vi "minicryo_SequenceRunner_202102.vi"() -> ()   [LabVIEW 2013]
uses:
  B_Globals.vi
  Global 2.vi
  DeltaRamp_globals.vi
panel:
  out "Output File":path=path "C:/User Data/Guang/EuS junction/EJJ 008D/JJ7_RH_8-10-14-1/RH_10uA_10K.txt"
  in  "Directory":path=path "C:/User Data/Guang/EuS junction/EJJ 008D/JJ7_RH_8-10-14-1"
  in  "T_high":dbl
  in  "T_low":dbl
  in  "Skip":bool
  out "Step":dbl
  out "Of":dbl=1.0
  out "Action":string="Waiting for go"
  in  "Start":bool
  in  "Array":T1(array[cluster])=[{"Combo Box"="Start R(H) (Bundle)", "Rate"=0.1, "Set Point"=-0.5, "String"="RH_10uA_10K", "Step [T]"=0.0, "Settle [s]"=0.0}]
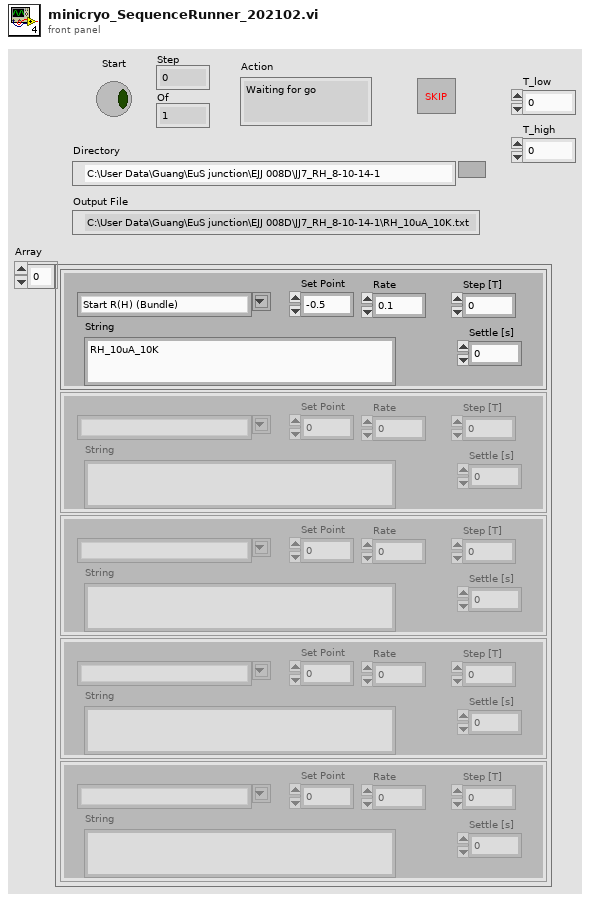
[diagram p1: front panel]
types:
  T1 = cluster{"Combo Box":string, "Rate":dbl, "Set Point":dbl, "String":string, "Step [T]":dbl, "Settle [s]":dbl}[]
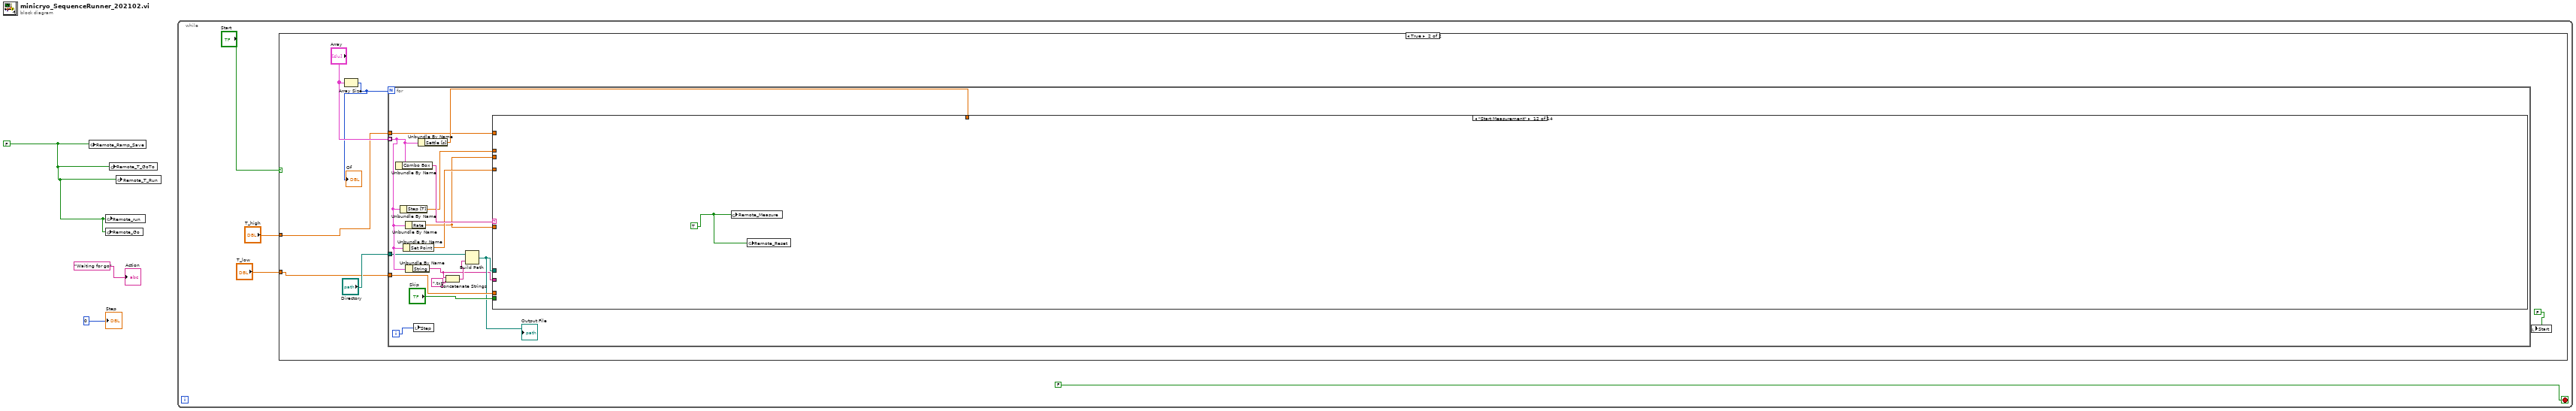
[diagram p0: block diagram]
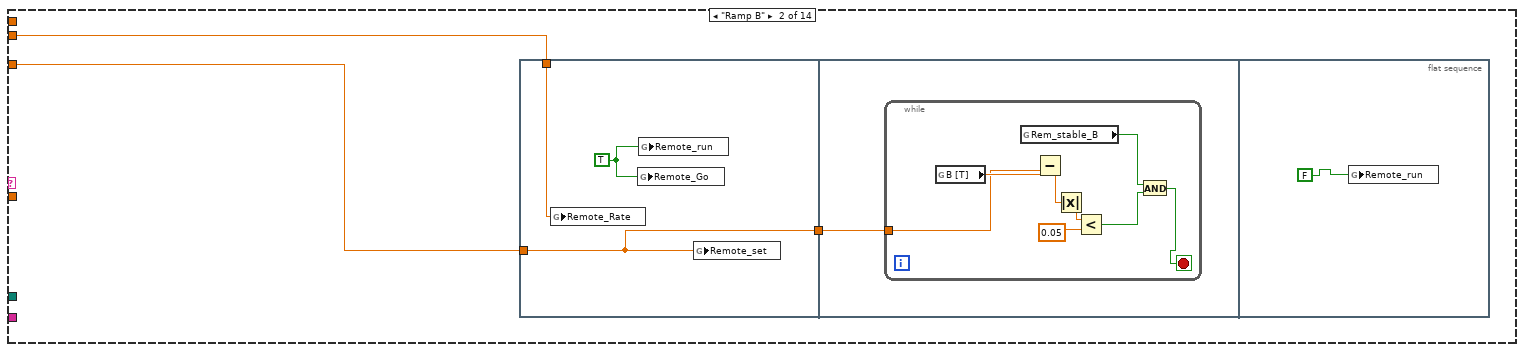
[diagram p4: hidden frame]
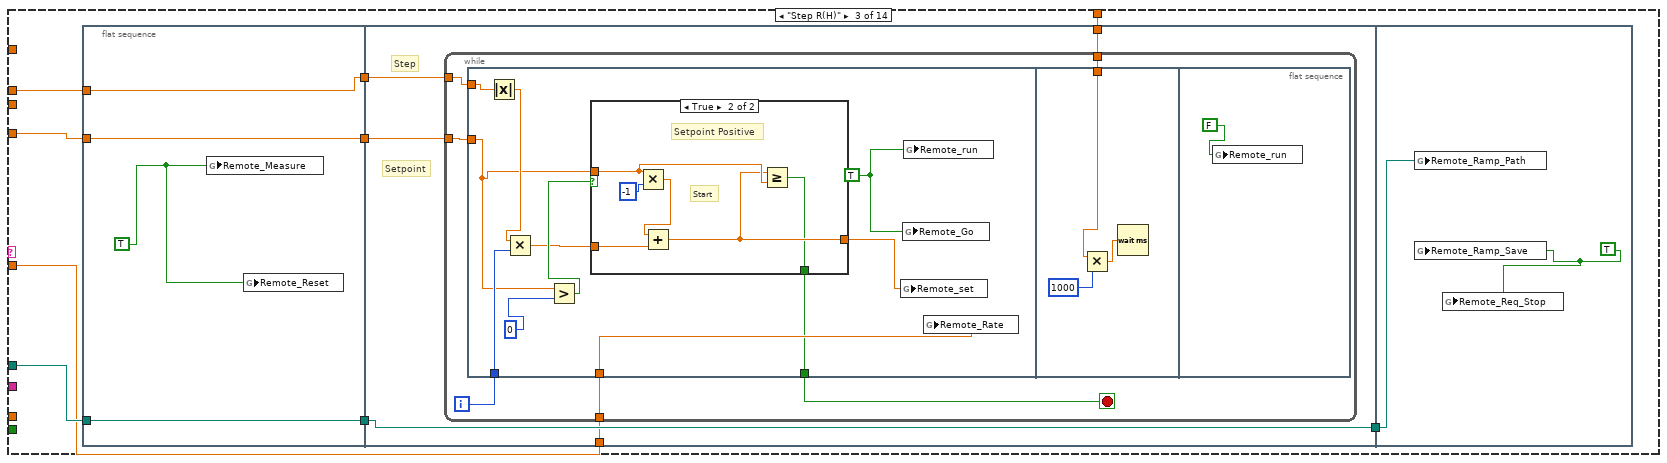
[diagram p5: hidden frame]
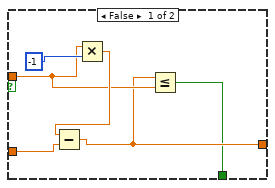
[diagram p6: hidden frame]
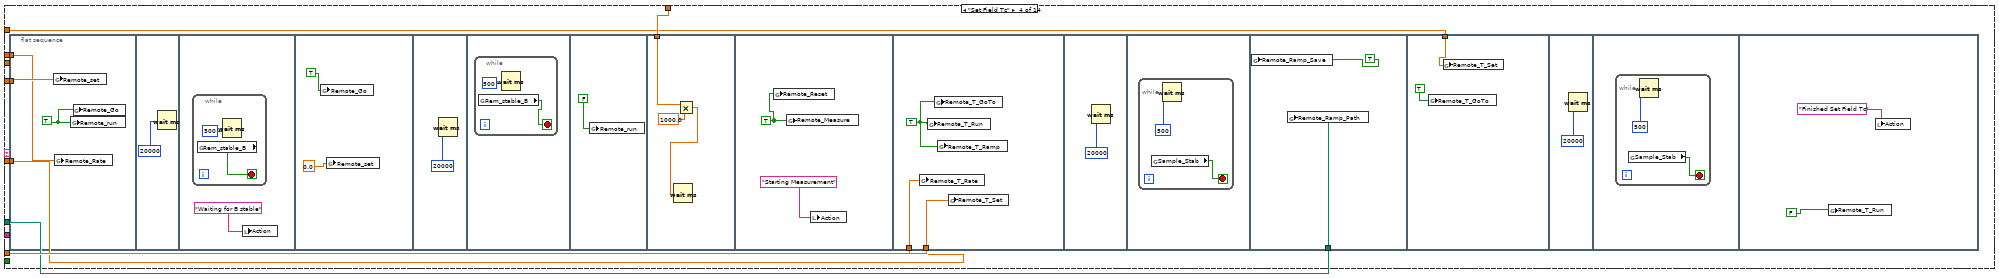
[diagram p7: hidden frame]
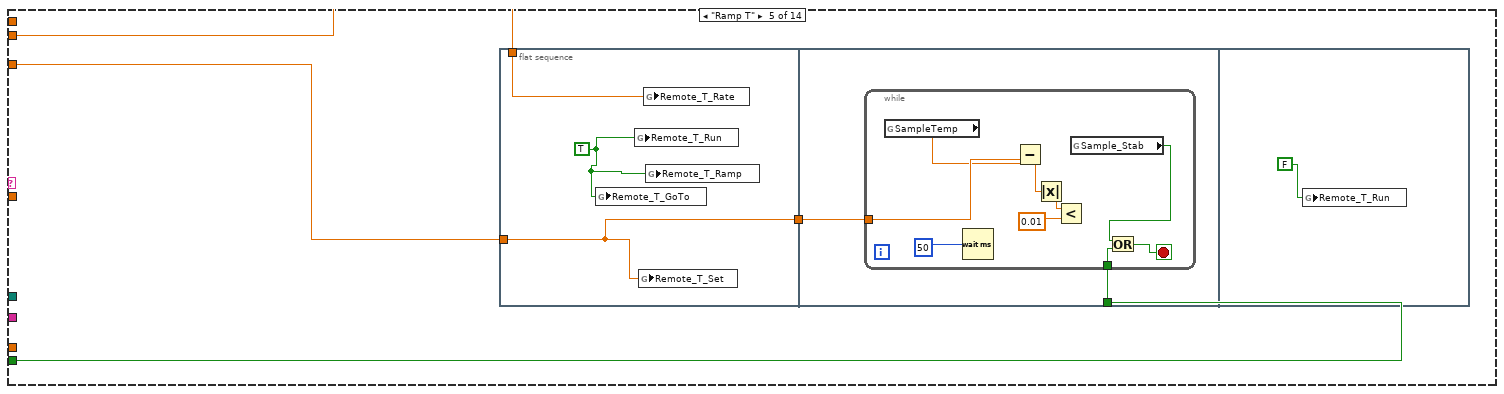
[diagram p8: hidden frame]
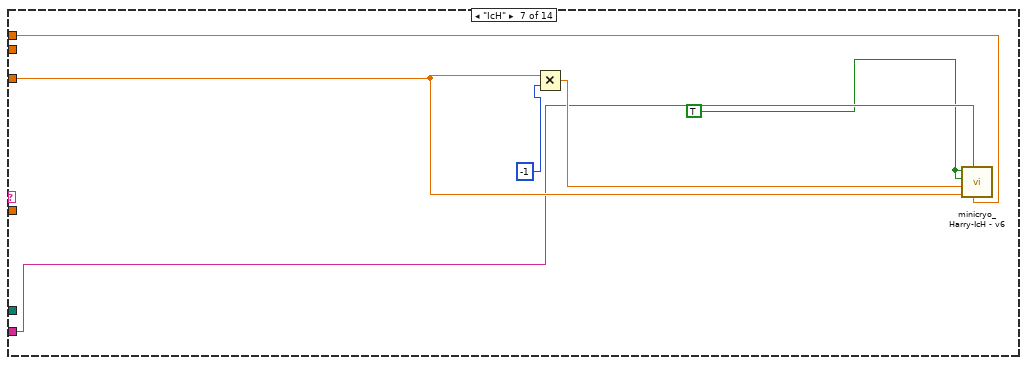
[diagram p10: hidden frame]
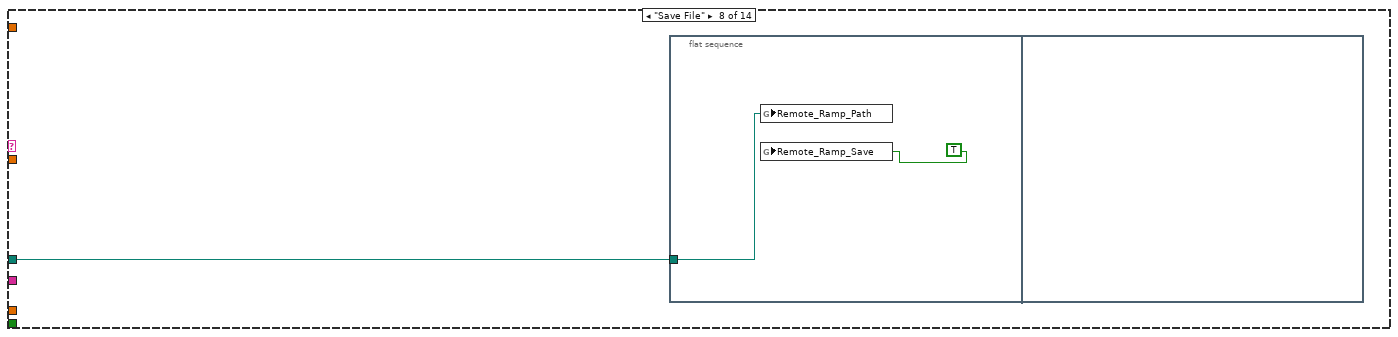
[diagram p11: hidden frame]
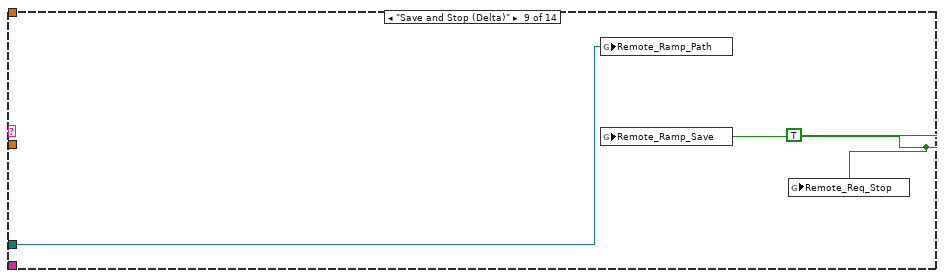
[diagram p12: hidden frame]
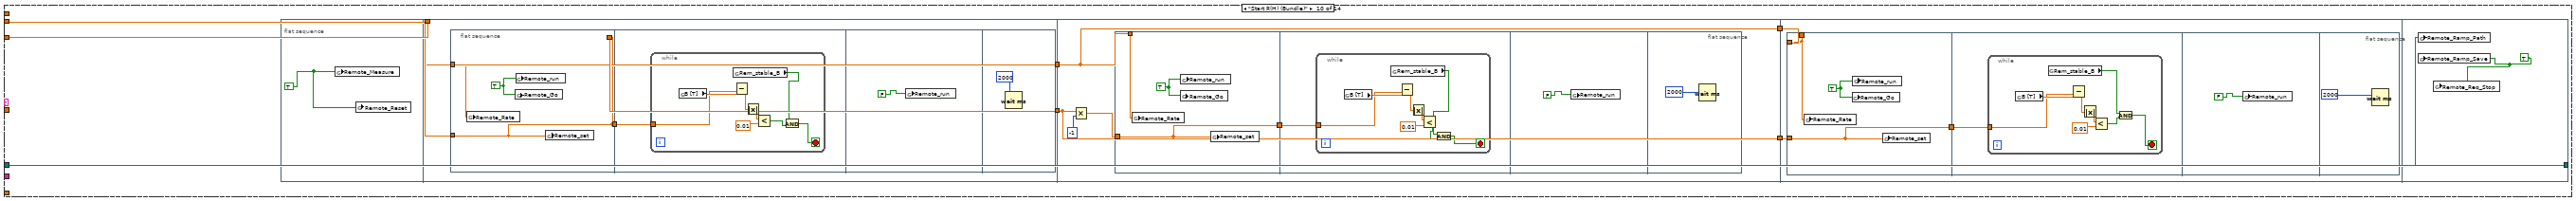
[diagram p13: hidden frame]
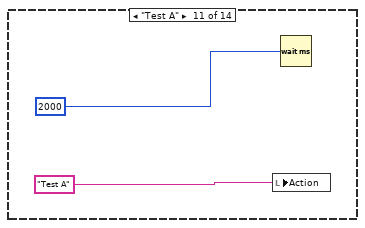
[diagram p14: hidden frame]
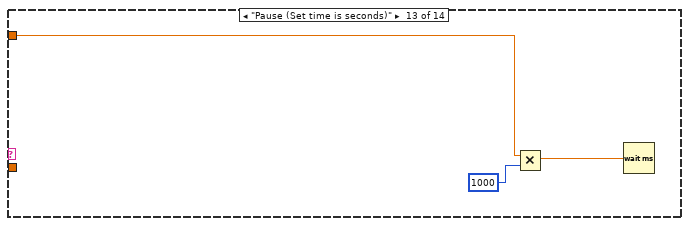
[diagram p15: hidden frame]
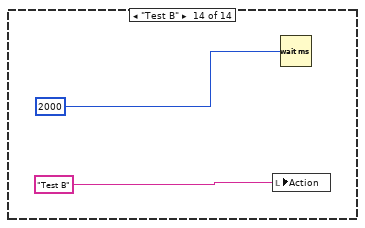
[diagram p16: hidden frame]
diagram:
  w3 = FALSE
  n1 = global write "DeltaRamp_globals.vi" "Remote_Ramp_Save"(w3) -> ()
  n2 = global write "B_Globals.vi" "Remote_Go"(w3) -> ()
  n3 = global write "B_Globals.vi" "Remote_run"(w3) -> ()
  n4 = global write "Global 2.vi" "Remote_T_GoTo"(w3) -> ()
  n5 = global write "Global 2.vi" "Remote_T_Run"(w3) -> ()
  n6 = while {
    stop <- FALSE stop-if-true
    n7 = case shown="True" "Start" {
      tunnel: "T_high" -> [_ w8]
      tunnel: "T_low" -> [_ w9]
      frame False {
      }
      frame True {
        n8 = Array Size(array="Array") -> (size(s)=w11:i32)
        "Of" <- w11
        n9 = for {
          N: w11 -> [_]
          tunnel: "Array" -> [w24] mode=indexing
          tunnel: "Directory" -> [w20]
          tunnel: w9 -> [w17]
          tunnel: w8 -> [w16]
          i -> [w26]
          n10 = Unbundle By Name(w24) -> ("Combo Box"=w28:string)
          n11 = Unbundle By Name(w24) -> ("Step [T]"=w22:dbl)
          n12 = Unbundle By Name(w24) -> ("Set Point"=w27:dbl)
          n13 = Unbundle By Name(w24) -> ("Rate"=w21:dbl)
          n14 = Unbundle By Name(w24) -> ("String"=w14:string)
          n15 = local write "Step"(w26) -> ()
          n16 = Unbundle By Name(w24) -> ("Settle [s]"=w23:dbl)
          n17 = Concatenate Strings(w14, ".txt") -> (w18:string)
          n18 = Build Path(base path=w20, name or relative path=w18) -> (appended path=w15:path)
          "Output File" <- w15
          n19 = case shown="\"Start Measurement\"" w28 {
            tunnel: w27 -> [_ w31 w49 w104 w139 _ w160 _ _ w174 _ _ w236 _]
            tunnel: w21 -> [_ w30 _ _ w140 _ _ _ _ w173 _ _ _ _]
            tunnel: w15 -> [_ _ w52 w99 _ _ _ w163 w167 w168 _ _ _ _]
            tunnel: "Skip" -> [_ _ _ _ w138 _ _ _ _ _ _ _ _ _]
            tunnel: w23 -> [_ _ w47 w103 _ _ _ _ _ _ _ _ _ _]
            tunnel: w22 -> [_ _ w46 w98 _ _ w159 _ _ _ _ _ _ _]
            tunnel: w21 -> [_ _ w45 w101 _ _ _ _ _ _ _ _ _ _]
            tunnel: w17 -> [_ _ _ w102 _ _ _ _ _ _ _ _ _ _]
            tunnel: w16 -> [_ _ _ w100 _ _ _ _ _ _ _ _ _ _]
            tunnel: w14 -> [_ _ _ _ _ _ w158 _ _ _ _ _ _ _]
            frame "False", Default {
            }
            frame "Ramp B" {
              n20 = flat-sequence {
                tunnel: w31 -> [w32]
                tunnel: w30 -> [w33]
                tunnel: [w32] -> w29
                tunnel: w29 -> [w35]
                frame #0 {
                  w34 = TRUE
                  n21 = global write "B_Globals.vi" "Remote_Rate"(w33) -> ()
                  n22 = global write "B_Globals.vi" "Remote_Go"(w34) -> ()
                  n23 = global write "B_Globals.vi" "Remote_run"(w34) -> ()
                  n24 = global write "B_Globals.vi" "Remote_set"(w32) -> ()
                }
                frame #1 {
                  n25 = while {
                    tunnel: w35 -> [w42]
                    stop <- w36 stop-if-true
                    n26 = global read "B_Globals.vi" "B [T]"() -> (w43:dbl)
                    n27 = global read "B_Globals.vi" "Rem_stable_B"() -> (w38:bool)
                    n28 = Subtract(x=w43, y=w42) -> (x-y=w41:dbl)
                    n29 = Absolute Value(x=w41) -> (abs(x)=w40:dbl)
                    n30 = Less?(x=w40, y=0.05) -> (x < y?=w37:bool)
                    n31 = And(x=w38, y=w37) -> (x .and. y?=w36:bool)
                  }
                }
                frame #2 {
                  n32 = global write "B_Globals.vi" "Remote_run"(FALSE) -> ()
                }
              }
            }
            frame "Step R(H)" {
              n33 = flat-sequence {
                tunnel: [w56] -> w53
                tunnel: w52 -> [w56]
                tunnel: [w55] -> w50
                tunnel: w49 -> [w55]
                tunnel: [w54] -> w48
                tunnel: w46 -> [w54]
                tunnel: w53 -> [w62]
                tunnel: [w62] -> w51
                tunnel: w50 -> [w61]
                tunnel: w48 -> [w60]
                tunnel: w47 -> [w59]
                tunnel: w45 -> [w58]
                tunnel: w51 -> [w96]
                frame #0 {
                  w57 = TRUE
                  n34 = global write "DeltaRamp_globals.vi" "Remote_Measure"(w57) -> ()
                  n35 = global write "DeltaRamp_globals.vi" "Remote_Reset"(w57) -> ()
                }
                frame #1 {
                  # "Step"
                  # "Setpoint"
                  n36 = while {
                    tunnel: w61 -> [w68]
                    tunnel: w60 -> [w66]
                    tunnel: w59 -> [w65]
                    tunnel: w58 -> [w64]
                    i -> [w67]
                    stop <- w63 stop-if-true
                    n37 = flat-sequence {
                      tunnel: w68 -> [w72]
                      tunnel: w67 -> [w78]
                      tunnel: w66 -> [w76]
                      tunnel: w64 -> [w75]
                      tunnel: [w69] -> w63
                      tunnel: w65 -> [w94]
                      frame #0 {
                        w77 = TRUE
                        n38 = Absolute Value(x=w76) -> (abs(x)=w79:dbl)
                        n39 = Multiply(x=w79, y=w78) -> (x*y=w71:dbl)
                        n40 = Greater?(x=w72, y=0) -> (0:w73:bool)
                        n41 = case shown="True" w73 {
                          tunnel: w72 -> [w82 w88]
                          tunnel: w71 -> [w84 w89]
                          tunnel: [w81 w87] -> w70
                          tunnel: [w80 w86] -> w69
                          frame False {
                            n42 = Multiply(x=w82, y=-1) -> (x*y=w83:dbl)
                            n43 = Subtract(x=w83, y=w84) -> (x-y=w81:dbl)
                            n44 = Less Or Equal?(x=w81, y=w82) -> (x <= y?=w80:bool)
                          }
                          frame True {
                            # "Start"
                            # "Setpoint Positive"
                            n45 = Multiply(x=w88, y=-1) -> (x*y=w90:dbl)
                            n46 = Add(x=w90, y=w89) -> (x+y=w87:dbl)
                            n47 = Greater Or Equal?(x=w87, y=w88) -> (x >= y?=w86:bool)
                          }
                        }
                        n48 = global write "B_Globals.vi" "Remote_set"(w70) -> ()
                        n49 = global write "B_Globals.vi" "Remote_Go"(w77) -> ()
                        n50 = global write "B_Globals.vi" "Remote_run"(w77) -> ()
                        n51 = global write "B_Globals.vi" "Remote_Rate"(w75) -> ()
                      }
                      frame #1 {
                        n52 = Multiply(x=w94, y=1000) -> (x*y=w93:dbl)
                        n53 = Wait (ms)(milliseconds to wait=w93) -> ()  [unwired: 1 out]
                      }
                      frame #2 {
                        n54 = global write "B_Globals.vi" "Remote_run"(FALSE) -> ()
                      }
                    }
                  }
                }
                frame #2 {
                  w97 = TRUE
                  n55 = global write "DeltaRamp_globals.vi" "Remote_Ramp_Path"(w96) -> ()
                  n56 = global write "DeltaRamp_globals.vi" "Remote_Ramp_Save"(w97) -> ()
                  n57 = global write "DeltaRamp_globals.vi" "Remote_Req_Stop"(w97) -> ()
                }
              }
            }
            frame "Set Field Tc" {
              n58 = flat-sequence {
                tunnel: w104 -> [w106]
                tunnel: w101 -> [_]
                tunnel: w98 -> [w105]
                tunnel: w103 -> [w119]
                tunnel: w102 -> [w124]
                tunnel: w101 -> [w123]
                tunnel: w99 -> [w130]
                tunnel: w100 -> [w132]
                frame #0 {
                  w107 = TRUE
                  n59 = global write "B_Globals.vi" "Remote_set"(w106) -> ()
                  n60 = global write "B_Globals.vi" "Remote_Rate"(w105) -> ()
                  n61 = global write "B_Globals.vi" "Remote_run"(w107) -> ()
                  n62 = global write "B_Globals.vi" "Remote_Go"(w107) -> ()
                }
                frame #1 {
                  n63 = Wait (ms)(milliseconds to wait=20000) -> ()  [unwired: 1 out]
                }
                frame #2 {
                  n64 = while {
                    stop <- w110 stop-if-true
                    n65 = global read "B_Globals.vi" "Rem_stable_B"() -> (w110:bool)
                    n66 = Wait (ms)(milliseconds to wait=500) -> ()  [unwired: 1 out]
                  }
                  n67 = local write "Action"("Waiting for B stable") -> ()
                }
                frame #3 {
                  n68 = global write "B_Globals.vi" "Remote_Go"(TRUE) -> ()
                  n69 = global write "B_Globals.vi" "Remote_set"(0.0) -> ()
                }
                frame #4 {
                  n70 = Wait (ms)(milliseconds to wait=20000) -> ()  [unwired: 1 out]
                }
                frame #5 {
                  n71 = while {
                    stop <- w116 stop-if-true
                    n72 = global read "B_Globals.vi" "Rem_stable_B"() -> (w116:bool)
                    n73 = Wait (ms)(milliseconds to wait=500) -> ()  [unwired: 1 out]
                  }
                }
                frame #6 {
                  n74 = global write "B_Globals.vi" "Remote_run"(FALSE) -> ()
                }
                frame #7 {
                  n75 = Multiply(x=w119, y=1000.0) -> (x*y=w118:dbl)
                  n76 = Wait (ms)(milliseconds to wait=w118) -> ()  [unwired: 1 out]
                }
                frame #8 {
                  w122 = TRUE
                  n77 = global write "DeltaRamp_globals.vi" "Remote_Reset"(w122) -> ()
                  n78 = global write "DeltaRamp_globals.vi" "Remote_Measure"(w122) -> ()
                  n79 = local write "Action"("Starting Measurement") -> ()
                }
                frame #9 {
                  w125 = TRUE
                  n80 = global write "Global 2.vi" "Remote_T_Rate"(w123) -> ()
                  n81 = global write "Global 2.vi" "Remote_T_Run"(w125) -> ()
                  n82 = global write "Global 2.vi" "Remote_T_GoTo"(w125) -> ()
                  n83 = global write "Global 2.vi" "Remote_T_Ramp"(w125) -> ()
                  n84 = global write "Global 2.vi" "Remote_T_Set"(w124) -> ()
                }
                frame #10 {
                  n85 = Wait (ms)(milliseconds to wait=20000) -> ()  [unwired: 1 out]
                }
                frame #11 {
                  n86 = while {
                    stop <- w128 stop-if-true
                    n87 = global read "Global 2.vi" "Sample_Stab"() -> (w128:bool)
                    n88 = Wait (ms)(milliseconds to wait=500) -> ()  [unwired: 1 out]
                  }
                }
                frame #12 {
                  n89 = global write "DeltaRamp_globals.vi" "Remote_Ramp_Save"(TRUE) -> ()
                  n90 = global write "DeltaRamp_globals.vi" "Remote_Ramp_Path"(w130) -> ()
                }
                frame #13 {
                  n91 = global write "Global 2.vi" "Remote_T_GoTo"(TRUE) -> ()
                  n92 = global write "Global 2.vi" "Remote_T_Set"(w132) -> ()
                }
                frame #14 {
                  n93 = Wait (ms)(milliseconds to wait=20000) -> ()  [unwired: 1 out]
                }
                frame #15 {
                  n94 = while {
                    stop <- w135 stop-if-true
                    n95 = global read "Global 2.vi" "Sample_Stab"() -> (w135:bool)
                    n96 = Wait (ms)(milliseconds to wait=500) -> ()  [unwired: 1 out]
                  }
                }
                frame #16 {
                  n97 = global write "Global 2.vi" "Remote_T_Run"(FALSE) -> ()
                  n98 = local write "Action"("Finished Set Field Tc") -> ()
                }
              }
            }
            frame "Ramp T" {
              n99 = flat-sequence {
                tunnel: w139 -> [w143]
                tunnel: [w143] -> w141
                tunnel: w140 -> [w144]
                tunnel: w141 -> [w146]
                tunnel: w138 -> [w145]
                frame #0 {
                  w142 = TRUE
                  n100 = global write "Global 2.vi" "Remote_T_GoTo"(w142) -> ()
                  n101 = global write "Global 2.vi" "Remote_T_Run"(w142) -> ()
                  n102 = global write "Global 2.vi" "Remote_T_Set"(w143) -> ()
                  n103 = global write "Global 2.vi" "Remote_T_Rate"(w144) -> ()
                  n104 = global write "Global 2.vi" "Remote_T_Ramp"(w142) -> ()
                }
                frame #1 {
                  n105 = while {
                    tunnel: w146 -> [w155]
                    tunnel: w145 -> [w149]
                    stop <- w150 stop-if-true
                    n106 = global read "Global 2.vi" "SampleTemp"() -> (w151:dbl)
                    n107 = Wait (ms)(milliseconds to wait=50) -> ()  [unwired: 1 out]
                    n108 = Subtract(x=w151, y=w155) -> (x-y=w154:dbl)
                    n109 = Absolute Value(x=w154) -> (abs(x)=w153:dbl)
                    n110 = Less?(x=w153, y=0.01) -> ()  [unwired: 1 out]
                    n111 = global read "Global 2.vi" "Sample_Stab"() -> (w148:bool)
                    n112 = Or(x=w148, y=w149) -> (x .or. y?=w150:bool)
                  }
                }
                frame #2 {
                  n113 = global write "Global 2.vi" "Remote_T_Run"(FALSE) -> ()
                }
              }
            }
            frame "Start R(T) (Bundle)" {
            }
            frame "IcH" {
              w157 = TRUE
              n114 = Multiply(x=w160, y=-1) -> (x*y=w161:dbl)
              n115 = call "minicryo_Harry-IcH - v6.vi"("Mag Field Step"=w159, "Directory Output"=w158, "Stop Field"=w160, "Start Field (T)"=w161, "Stop"=w157, "Measure"=w157) -> ()  [unwired: 6 in]
            }
            frame "Save File" {
              n116 = flat-sequence {
                tunnel: w163 -> [w165]
                frame #0 {
                  n117 = global write "DeltaRamp_globals.vi" "Remote_Ramp_Path"(w165) -> ()
                  n118 = global write "DeltaRamp_globals.vi" "Remote_Ramp_Save"(TRUE) -> ()
                }
                frame #1 {
                }
              }
            }
            frame "Save and Stop (Delta)" {
              w166 = TRUE
              n119 = global write "DeltaRamp_globals.vi" "Remote_Ramp_Path"(w167) -> ()
              n120 = global write "DeltaRamp_globals.vi" "Remote_Ramp_Save"(w166) -> ()
              n121 = global write "DeltaRamp_globals.vi" "Remote_Req_Stop"(w166) -> ()
            }
            frame "Start R(H) (Bundle)" {
              n122 = flat-sequence {
                tunnel: w174 -> [w178]
                tunnel: w173 -> [w176]
                tunnel: [w177] -> w172
                tunnel: [w176] -> w171
                tunnel: w172 -> [w194]
                tunnel: w171 -> [w195]
                tunnel: [w195] -> w170
                tunnel: [w194] -> w169
                tunnel: w170 -> [w214]
                tunnel: w169 -> [w213]
                tunnel: w168 -> [w230]
                frame #0 {
                  w175 = TRUE
                  n123 = global write "DeltaRamp_globals.vi" "Remote_Measure"(w175) -> ()
                  n124 = global write "DeltaRamp_globals.vi" "Remote_Reset"(w175) -> ()
                }
                frame #1 {
                  n125 = flat-sequence {
                    tunnel: w178 -> [w180]
                    tunnel: [w180] -> w179
                    tunnel: w176 -> [w181]
                    tunnel: [w180] -> w177
                    tunnel: w179 -> [w183]
                    frame #0 {
                      w182 = TRUE
                      n126 = global write "B_Globals.vi" "Remote_Rate"(w181) -> ()
                      n127 = global write "B_Globals.vi" "Remote_Go"(w182) -> ()
                      n128 = global write "B_Globals.vi" "Remote_run"(w182) -> ()
                      n129 = global write "B_Globals.vi" "Remote_set"(w180) -> ()
                    }
                    frame #1 {
                      n130 = while {
                        tunnel: w183 -> [w190]
                        stop <- w184 stop-if-true
                        n131 = global read "B_Globals.vi" "B [T]"() -> (w191:dbl)
                        n132 = global read "B_Globals.vi" "Rem_stable_B"() -> (w185:bool)
                        n133 = Subtract(x=w191, y=w190) -> (x-y=w189:dbl)
                        n134 = Absolute Value(x=w189) -> (abs(x)=w188:dbl)
                        n135 = Less?(x=w188, y=0.01) -> (x < y?=w186:bool)
                        n136 = And(x=w185, y=w186) -> (x .and. y?=w184:bool)
                      }
                    }
                    frame #2 {
                      n137 = global write "B_Globals.vi" "Remote_run"(FALSE) -> ()
                    }
                    frame #3 {
                      n138 = Wait (ms)(milliseconds to wait=2000) -> ()  [unwired: 1 out]
                    }
                  }
                }
                frame #2 {
                  n139 = Multiply(x=w194, y=-1) -> (x*y=w196:dbl)
                  n140 = flat-sequence {
                    tunnel: w196 -> [w199]
                    tunnel: w195 -> [w200]
                    tunnel: [w199] -> w198
                    tunnel: w198 -> [w202]
                    frame #0 {
                      w201 = TRUE
                      n141 = global write "B_Globals.vi" "Remote_Rate"(w200) -> ()
                      n142 = global write "B_Globals.vi" "Remote_Go"(w201) -> ()
                      n143 = global write "B_Globals.vi" "Remote_run"(w201) -> ()
                      n144 = global write "B_Globals.vi" "Remote_set"(w199) -> ()
                    }
                    frame #1 {
                      n145 = while {
                        tunnel: w202 -> [w209]
                        stop <- w203 stop-if-true
                        n146 = global read "B_Globals.vi" "B [T]"() -> (w210:dbl)
                        n147 = global read "B_Globals.vi" "Rem_stable_B"() -> (w205:bool)
                        n148 = Subtract(x=w210, y=w209) -> (x-y=w208:dbl)
                        n149 = Absolute Value(x=w208) -> (abs(x)=w207:dbl)
                        n150 = Less?(x=w207, y=0.01) -> (x < y?=w204:bool)
                        n151 = And(x=w205, y=w204) -> (x .and. y?=w203:bool)
                      }
                    }
                    frame #2 {
                      n152 = global write "B_Globals.vi" "Remote_run"(FALSE) -> ()
                    }
                    frame #3 {
                      n153 = Wait (ms)(milliseconds to wait=2000) -> ()  [unwired: 1 out]
                    }
                  }
                }
                frame #3 {
                  n154 = flat-sequence {
                    tunnel: w213 -> [w217]
                    tunnel: [w216] -> _
                    tunnel: [w217] -> w215
                    tunnel: w214 -> [w216]
                    tunnel: w215 -> [w219]
                    frame #0 {
                      w218 = TRUE
                      n155 = global write "B_Globals.vi" "Remote_Rate"(w216) -> ()
                      n156 = global write "B_Globals.vi" "Remote_Go"(w218) -> ()
                      n157 = global write "B_Globals.vi" "Remote_run"(w218) -> ()
                      n158 = global write "B_Globals.vi" "Remote_set"(w217) -> ()
                    }
                    frame #1 {
                      n159 = while {
                        tunnel: w219 -> [w226]
                        stop <- w221 stop-if-true
                        n160 = global read "B_Globals.vi" "B [T]"() -> (w227:dbl)
                        n161 = global read "B_Globals.vi" "Rem_stable_B"() -> (w220:bool)
                        n162 = Subtract(x=w227, y=w226) -> (x-y=w225:dbl)
                        n163 = Absolute Value(x=w225) -> (abs(x)=w224:dbl)
                        n164 = Less?(x=w224, y=0.01) -> (x < y?=w222:bool)
                        n165 = And(x=w220, y=w222) -> (x .and. y?=w221:bool)
                      }
                    }
                    frame #2 {
                      n166 = global write "B_Globals.vi" "Remote_run"(FALSE) -> ()
                    }
                    frame #3 {
                      n167 = Wait (ms)(milliseconds to wait=2000) -> ()  [unwired: 1 out]
                    }
                  }
                }
                frame #4 {
                  w231 = TRUE
                  n168 = global write "DeltaRamp_globals.vi" "Remote_Ramp_Path"(w230) -> ()
                  n169 = global write "DeltaRamp_globals.vi" "Remote_Ramp_Save"(w231) -> ()
                  n170 = global write "DeltaRamp_globals.vi" "Remote_Req_Stop"(w231) -> ()
                }
              }
            }
            frame "Test A" {
              n171 = local write "Action"("Test A") -> ()
              n172 = Wait (ms)(milliseconds to wait=2000) -> ()  [unwired: 1 out]
            }
            frame "Start Measurement" {
              w234 = TRUE
              n173 = global write "DeltaRamp_globals.vi" "Remote_Measure"(w234) -> ()
              n174 = global write "DeltaRamp_globals.vi" "Remote_Reset"(w234) -> ()
            }
            frame "Pause (Set time is seconds)" {
              n175 = Multiply(x=w236, y=1000) -> (x*y=w235:dbl)
              n176 = Wait (ms)(milliseconds to wait=w235) -> ()  [unwired: 1 out]
            }
            frame "Test B" {
              n177 = local write "Action"("Test B") -> ()
              n178 = Wait (ms)(milliseconds to wait=2000) -> ()  [unwired: 1 out]
            }
          }
        }
        n179 = local write "Start"(FALSE) -> ()
      }
    }
  }
  "Action" <- "Waiting for go"
  "Step" <- 0
